vi "Global dati tab freddo.vi"() -> ()   [LabVIEW 2019]
panel:
  out "dati tab freddo":bool
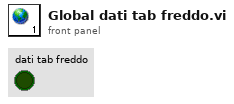
[diagram p1: front panel]
diagram:
